vi "Master_Initializer.vi"(8 "error in (no error)":errorcluster, 10 "FPGA VI Reference In":refnum<k20>) -> (0 "error out":errorcluster, 2 "FPGA VI Reference Out":refnum<k20>)   [LabVIEW 2018]
doc: "Ensures all outputs and variables are set to a safe value (FALSE for most), prior to running the rest of the VI. If values cannot be set for any reason, an error will be given, after a 10 second timeout."
uses:
  DAQ/Master_DataControl.ctl
  DAQ/TypeDef_cRIOData.ctl
  IMU/TypeDef_IMUData.ctl
  CAN/TypeDef_BMSData.ctl
  CAN/TypeDef_BMS_Status.ctl
  CAN/MotorController/fixedMotorData.ctl
  CAN/MotorController/MotorStatus.ctl
  Host/Libraries/TypeDef_CurrentState.ctl
  TypeDef_LoopPeriods.ctl
  <vilib>/Utility/error.llb/Error Cluster From Error Code.vi
  <vilib>/rvi/errors/niLvFpgaAdjustHostInterfaceError.vi
  <vilib>/rvi/interface/nirviReadWriteControl/nirviReadWriteControl.xnode
  <vilib>/NI_Real-Time Target Support.lvlib
  NiFpgaLv.dll
  <vilib>/rvi/interface/Simulation/niFpgaSimulationCallBeginRW.vi
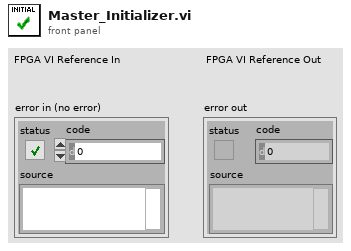
[diagram p1: front panel]
types:
  T1 = typedef "TypeDef_BMSData.ctl" = cluster{"Max Cell Voltage (V)":dbl, "Max Cell ID":dbl, "Min Cell Voltage (V)":dbl, "Min Cell ID":dbl, "State of Charge (%)":dbl, "Average Voltage (V)":dbl, "Voltage Delta (V)":dbl, "Pack Current (A)":dbl, "Pack Voltage (V)":dbl, "Max Resistance (Ohm)":dbl, "Min Resistance (Ohm)":dbl, "Average Resistance (Ohm)":dbl, "Delta Resistance (Ohm)":dbl, "Highest Temperature(F)":dbl, "BmsStatus":T2}
  T2 = typedef "TypeDef_BMS_Status.ctl" = cluster{"isFault":bool, "isolationMonitoring":bool}
  T3 = typedef "TypeDef_CurrentState.ctl" = enum16{"Fault", "Idle", "Ready", "Pushing", "Coast", "Braking"}
  T4 = typedef "Master_DataControl.ctl" = cluster{"cRIO Data":T5, "IMU Data":T6, "BMS Data":T1, "Motor Data":T7}
  T5 = typedef "TypeDef_cRIOData.ctl" = cluster{"Time (ms)":dbl, "24V Battery (V)":dbl, "LowV Current (A)":dbl, "Fiducial Sensor (V)":dbl, "PV Pressure (psig)":dbl, "Flow Sensor (V)":dbl, "Temp Fairing (F)":dbl, "Temp Reservoir (F)":dbl, "HallEffect Right (in)":dbl, "HallEffect Left (in)":dbl, "PT Tank (psig)":dbl, "PT Clamp Right (psig)":dbl, "PT Clamp Left (psig)":dbl, "PT Brake (psig)":dbl, "PT Cooling (psig)":dbl, "Displacement (ft)":dbl, "Velocity (ft/s)":dbl}
  T6 = typedef "TypeDef_IMUData.ctl" = cluster{"x acceleration (g)":dbl, "Pressure (psia)":dbl, "Temperature (F)":dbl}
  T7 = typedef "fixedMotorData.ctl" = cluster{"Velo (RPM)":dbl, "MotorTemp(F)":dbl, "CtrlTemp(F)":dbl, "DcLinkVolt(V)":dbl, "ErrorCode":dbl, "motorStatus":T8, "isAlive":bool, "motorControllerState":u16}
  T8 = typedef "MotorStatus.ctl" = cluster{"isReady":bool, "isOn":bool, "isOperEn":bool, "isFault":bool, "isVoltEn":bool, "targetReached":bool, "isWarning":bool}
  T9 = typedef "TypeDef_LoopPeriods.ctl" = cluster{"Control Period":i64, "DAQ Period":u32, "IMU Period":u32, "CAN Period":i64, "Nav Period":u32}
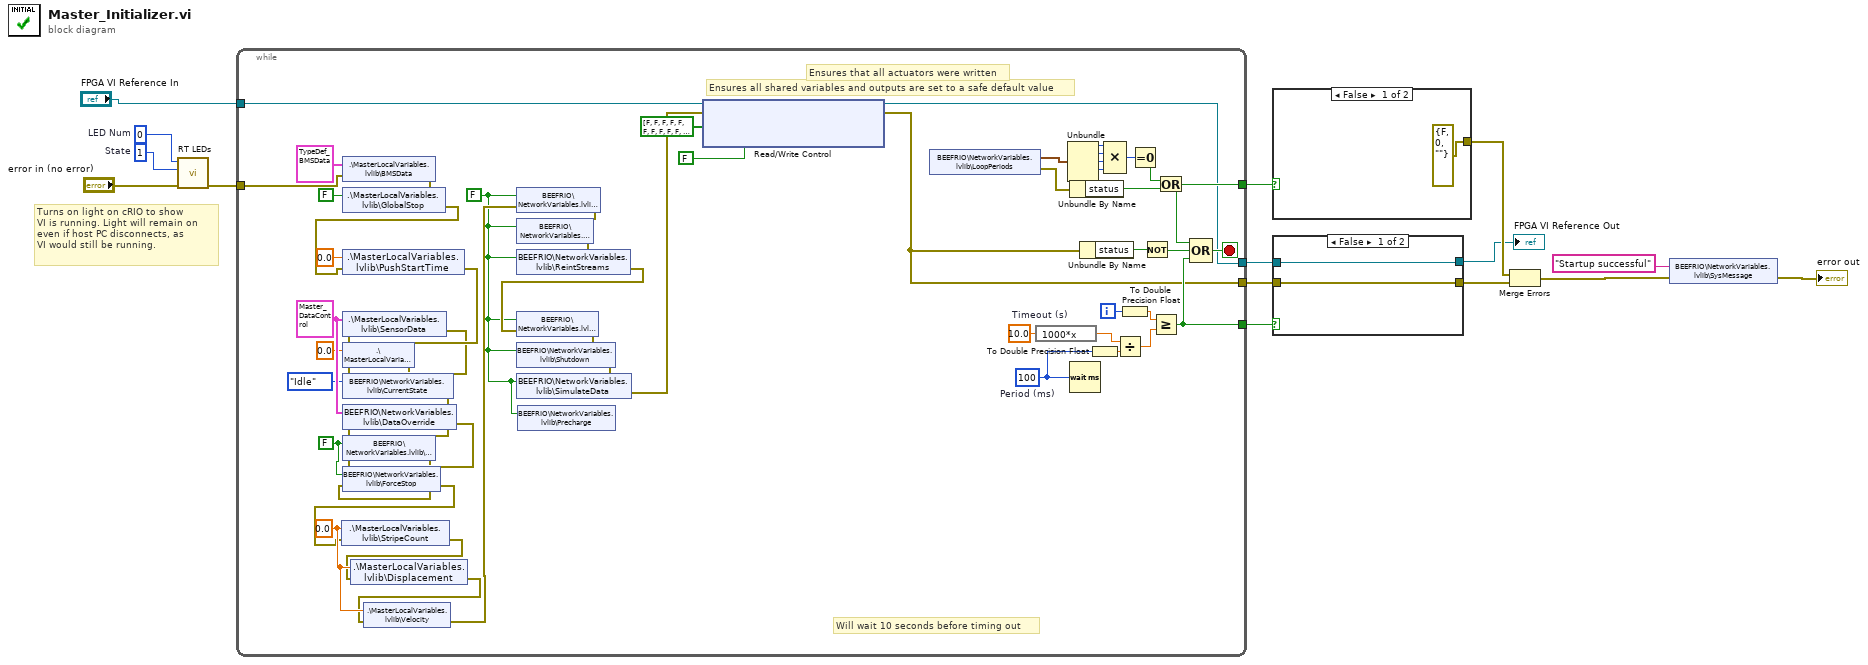
[diagram p0: block diagram]
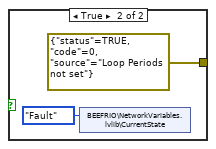
[diagram p2: hidden frame]
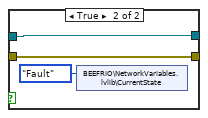
[diagram p3: hidden frame]
diagram:
  w10 = 0  # LED Num
  w9 = 1  # State
  # "Turns on light on cRIO to show\nVI is running. Light will remain on \neven if host PC disconnects, as \nVI would still be running."
  n1 = call <vilib>:"RT LEDs.vi"("error in (no error)"="error in (no error)", "State"=w9, "LED Num"=w10) -> ("error out"=w12:errorcluster)  [unwired: 3 in, 1 out]
  n2 = while {
    tunnel: [w45] -> w15
    tunnel: [w26] -> w14
    tunnel: w12 -> [w28]
    tunnel: [w29] -> w13
    tunnel: "FPGA VI Reference In" -> [w25]
    tunnel: [w24] -> w3
    i -> [w46]
    stop <- w68 stop-if-true
    w22 = 0.0 ("StripeCount")
    w44 = 10.0  # Timeout (s)
    w50 = FALSE ("ForceIdle")
    w53 = T4 {"cRIO Data"={"Time (ms)"=0.0, "24V Battery (V)"=0.0, "LowV Current (A)"=0.0, "Fiducial Sensor (V)"=0.0, "PV Pressure (psig)"=0.0, "Flow Sensor (V)"=0.0, "Temp Fairing (F)"=0.0, "Temp Reservoir (F)"=0.0, "HallEffect Right (in)"=0.0, "HallEffect Left (in)"=0.0, "PT Tank (psig)"=0.0, "PT Clamp Right (psig)"=0.0, "PT Clamp Left (psig)"=0.0, "PT Brake (psig)"=0.0, "PT Cooling (psig)"=0.0, "Displacement (ft)"=0.0, "Velocity (ft/s)"=0.0}, "IMU Data"={"x acceleration (g)"=0.0, "Pressure (psia)"=0.0, "Temperature (F)"=0.0}, "BMS Data"={"Max Cell Voltage (V)"=0.0, "Max Cell ID"=0.0, "Min Cell Voltage (V)"=0.0, "Min Cell ID"=0.0, "State of Charge (%)"=0.0, "Average Voltage (V)"=0.0, "Voltage Delta (V)"=0.0, "Pack Current (A)"=0.0, "Pack Voltage (V)"=0.0, "Max Resistance (Ohm)"=0.0, "Min Resistance (Ohm)"=0.0, "Average Resistance (Ohm)"=0.0, "Delta Resistance (Ohm)"=0.0, "Highest Temperature(F)"=0.0, "BmsStatus"={"isFault"=FALSE, "isolationMonitoring"=FALSE}}, "Motor Data"={"Velo (RPM)"=0.0, "MotorTemp(F)"=0.0, "CtrlTemp(F)"=0.0, "DcLinkVolt(V)"=0.0, "ErrorCode"=0.0, "motorStatus"={"isReady"=FALSE, "isOn"=FALSE, "isOperEn"=FALSE, "isFault"=FALSE, "isVoltEn"=FALSE, "targetReached"=FALSE, "isWarning"=FALSE}, "isAlive"=FALSE, "motorControllerState"=1}} ("SensorData")
    w17 = FALSE ("DumpValve")
    w42 = u32 100  # Period (ms)
    # "Will wait 10 seconds before timing out"
    # "Ensures that all actuators were written"
    # "Ensures all shared variables and outputs are set to a safe default value"
    n3 = shared-variable ".\\MasterLocalVariables.lvlib\\BMSData"(T1 {"Max Cell Voltage (V)"=0.0, "Max Cell ID"=0.0, "Min Cell Voltage (V)"=0.0, "Min Cell ID"=0.0, "State of Charge (%)"=0.0, "Average Voltage (V)"=0.0, "Voltage Delta (V)"=0.0, "Pack Current (A)"=0.0, "Pack Voltage (V)"=0.0, "Max Resistance (Ohm)"=0.0, "Min Resistance (Ohm)"=0.0, "Average Resistance (Ohm)"=0.0, "Delta Resistance (Ohm)"=0.0, "Highest Temperature(F)"=0.0, "BmsStatus"={"isFault"=FALSE, "isolationMonitoring"=FALSE}} ("CANData"), error in=w28) -> (error out=w66:errorcluster)
    n4 = shared-variable ".\\MasterLocalVariables.lvlib\\GlobalStop"(FALSE ("GlobalStop"), error in=w66) -> (error out=w65:errorcluster)
    n5 = shared-variable ".\\MasterLocalVariables.lvlib\\PushStartTime"(0.0 ("PushStartTime"), error in=w65) -> (error out=w64:errorcluster)
    n6 = shared-variable ".\\MasterLocalVariables.lvlib\\SensorData"(w53, error in=w64) -> (error out=w63:errorcluster)
    n7 = shared-variable ".\\MasterLocalVariables.lvlib\\Time"(0.0 ("Time"), error in=w63) -> (error out=w49:errorcluster)
    n8 = shared-variable "BEEFRIO\\NetworkVariables.lvlib\\CurrentState"(TypeDef_CurrentState."Idle" ("CurrentState"), error in=w49) -> (error out=w48:errorcluster)
    n9 = shared-variable "BEEFRIO\\NetworkVariables.lvlib\\DataOverride"(w53, error in=w48) -> (error out=w62:errorcluster)
    n10 = shared-variable "BEEFRIO\\NetworkVariables.lvlib\\ForceIdle"(w50, error in=w62) -> (error out=w61:errorcluster)
    n11 = shared-variable "BEEFRIO\\NetworkVariables.lvlib\\ForceStop"(w50, error in=w61) -> (error out=w19:errorcluster)
    n12 = shared-variable ".\\MasterLocalVariables.lvlib\\StripeCount"(w22, error in=w19) -> (error out=w21:errorcluster)
    n13 = shared-variable ".\\MasterLocalVariables.lvlib\\Displacement"(w22, error in=w21) -> (error out=w20:errorcluster)
    n14 = shared-variable ".\\MasterLocalVariables.lvlib\\Velocity"(w22, error in=w20) -> (error out=w18:errorcluster)
    n15 = shared-variable "BEEFRIO\\NetworkVariables.lvlib\\Launch"(w17, error in=w18) -> (error out=w60:errorcluster)
    n16 = shared-variable "BEEFRIO\\NetworkVariables.lvlib\\Ready"(w17, error in=w60) -> (error out=w59:errorcluster)
    n17 = shared-variable "BEEFRIO\\NetworkVariables.lvlib\\ReintStreams"(w17, error in=w59) -> (error out=w56:errorcluster)
    n18 = shared-variable "BEEFRIO\\NetworkVariables.lvlib\\Service"(w17, error in=w56) -> (error out=w58:errorcluster)
    n19 = shared-variable "BEEFRIO\\NetworkVariables.lvlib\\Shutdown"(w17, error in=w58) -> (error out=w57:errorcluster)
    n20 = shared-variable "BEEFRIO\\NetworkVariables.lvlib\\SimulateData"(w17, error in=w57) -> (error out=w27:errorcluster)
    n21 = shared-variable "BEEFRIO\\NetworkVariables.lvlib\\Precharge"(w17) -> ()  [unwired: 1 in, 1 out]
    n22 = xnode "Read/Write Control"("FPGA VI Reference In"=w25, "error in"=w27, "Digital Control Outputs"=bool[] [FALSE, FALSE, FALSE, FALSE, FALSE, FALSE, FALSE, FALSE, FALSE, FALSE, FALSE, FALSE, FALSE, FALSE, FALSE, FALSE], "RT Reset on Watchdog Failure?"=FALSE) -> ("FPGA VI Reference Out"=w24:refnum<k20>, "error out"=w26:errorcluster)
    n23 = shared-variable "BEEFRIO\\NetworkVariables.lvlib\\LoopPeriods"() -> (w38:T9, error out=w32:errorcluster)  [unwired: 1 in]
    n24 = expression code="1000*x"(w44) -> (w43:dbl)
    n25 = Unbundle(w38) -> ("Control Period"=w34:i64, "DAQ Period"=w36:u32, "IMU Period"=w35:u32, "CAN Period"=w37:i64)  [unwired: 1 out]
    n26 = Unbundle By Name(w32) -> ("status"=w30:bool)
    n27 = Wait (ms)(milliseconds to wait=w42) -> ()  [unwired: 1 out]
    n28 = Unbundle By Name(w26) -> ("status"=w69:bool)
    n29 = To Double Precision Float(number=w42) -> (double precision float=w40:dbl)
    n30 = Compound Arithmetic op=MULTIPLY(w34, w36, w35, w37) -> (w33:i64)
    n31 = Divide(x=w43, y=w40) -> (x/y=w41:dbl)
    n32 = To Double Precision Float(number=w46) -> (double precision float=w39:dbl)
    n33 = Equal To 0?(x=w33) -> (x = 0?=w31:bool)
    n34 = Not(x=w69) -> (.not. x?=w67:bool)
    n35 = Greater Or Equal?(x=w39, y=w41) -> (x >= y?=w45:bool)
    n36 = Or(x=w31, y=w30) -> (x .or. y?=w29:bool)
    n37 = Compound Arithmetic op=OR(w29, w67, w45) -> (w68:bool)
  }
  n38 = case shown="False" w13 {
    tunnel: [errorcluster {"status"=FALSE, "code"=0, "source"=""} ("error out") errorcluster {"status"=TRUE, "code"=0, "source"="Loop Periods not set"} ("error constant")] -> w7
    frame False {
    }
    frame True {
      n39 = shared-variable "BEEFRIO\\NetworkVariables.lvlib\\CurrentState"(TypeDef_CurrentState."Fault" ("Current State")) -> ()  [unwired: 1 in, 1 out]
    }
  }
  n40 = case shown="False" w15 {
    tunnel: [w73 w76] -> w8
    tunnel: w14 -> [w73 w76]
    tunnel: w3 -> [w74 w75]
    tunnel: [w74 w75] -> w1
    frame False {
    }
    frame True {
      n41 = shared-variable "BEEFRIO\\NetworkVariables.lvlib\\CurrentState"(TypeDef_CurrentState."Fault" ("Current State")) -> ()  [unwired: 1 in, 1 out]
    }
  }
  "FPGA VI Reference Out" <- w1
  n42 = Merge Errors(w7, w8) -> (w5:errorcluster)
  n43 = shared-variable "BEEFRIO\\NetworkVariables.lvlib\\SysMessage"("Startup successful" ("SysMessage"), error in=w5) -> (error out=→"error out":errorcluster)
